vi "Image Measure_mag.vi"() -> ()   [LabVIEW 2016]
panel:
  in  "Magnification":dbl(ring) items=["0.78"=2.01724e-06, "1.0"=1.57574e-06, "1.25"=1.256e-06, "1.6"=9.82138e-07, "2.0"=7.83072e-07, "2.5"=6.26894e-07, "3.2"=4.92295e-07, "4.0"=3.93809e-07, "5.0"=3.15056e-07, "6.3"=2.59e-07, "8.0"=2.079e-07, "10.0"=1.646e-07, "12.5"=1.33e-07, "16.0"=1.02e-07]
  out "Line length":dbl format="%#_6pm"
  out "Line pixel length":dbl
  out "Line":T1 {"Start X" scale=0.0..1024.0; "End X" scale=0.0..1024.0}
  out "ROI":T2
  out "Tool":i32(ring) items=["None", "Selection Tool", "Point Tool", "Line Tool", "Rectangle Tool", "Oval Tool", "Polygon Tool", "ClosedFreehandTool", "Annulus Tool", "Rotated Rectangle Tool", "Zoom Tool", "Pan Tool", "Polyline Tool", "Freehand Tool"]
  out "Type":i32(ring) items=["No Event"=0, "Click Event"=1, "Draw Event"=2, "Size Event"=4, "Scroll Event"=5, "Double Click Event"=8]
  in  "Stop Button":bool
  in  "Image  path":path
  out "Image":T3(plugin-control)
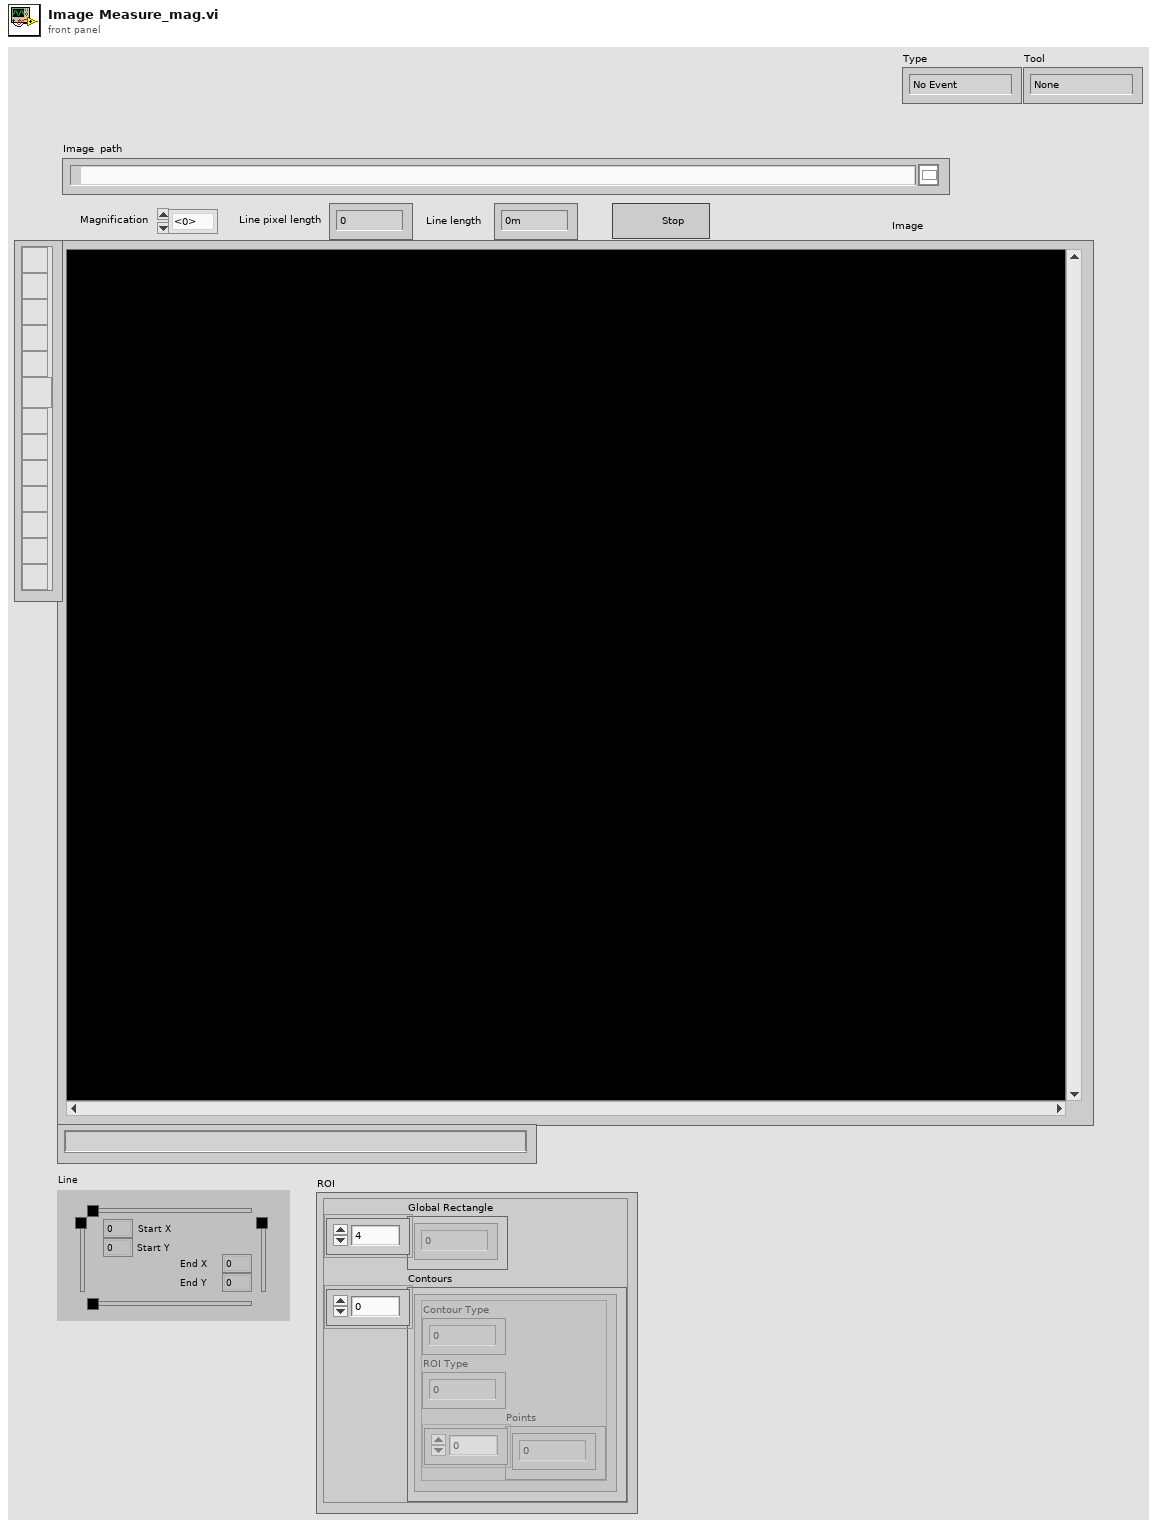
[diagram p1: front panel]
types:
  T1 = typedef "IMAQ Line" = cluster{"Start X":i32, "Start Y":i32, "End X":i32, "End Y":i32}
  T2 = cluster{"Global Rectangle":i32[], "Contours":cluster{"Contour Type":u32, "ROI Type":u32, "Points":i32[]}[]}
  T3 = typedef "IMAQ Image.ctl" = refnum<image>
  T4 = typedef "Image Type" = u32
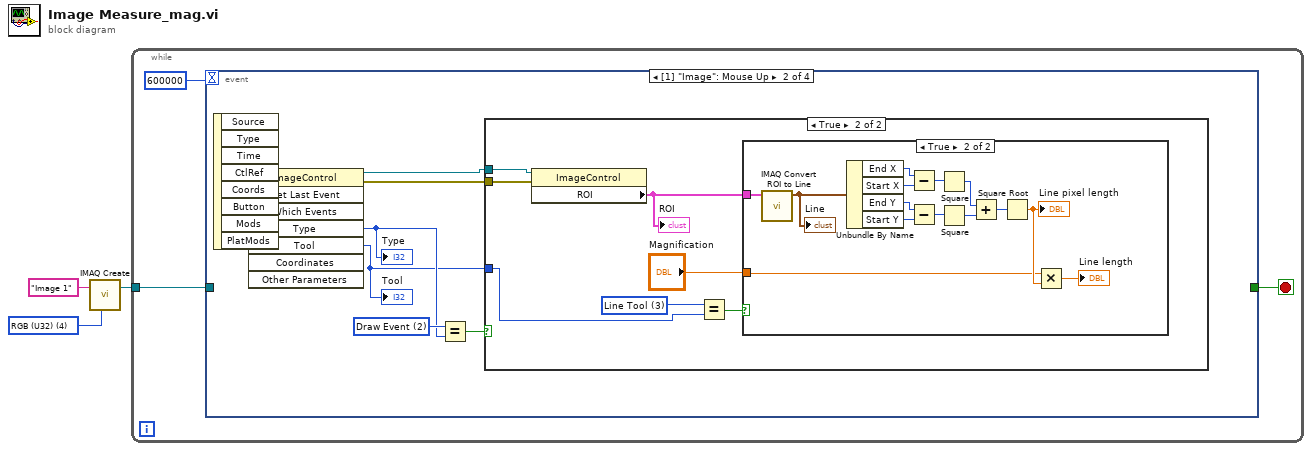
[diagram p0: block diagram]
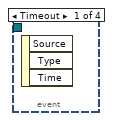
[diagram p2: hidden frame]
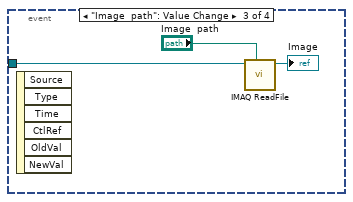
[diagram p5: hidden frame]
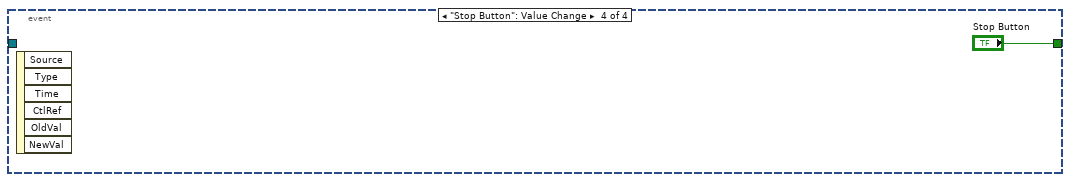
[diagram p6: hidden frame]
diagram:
  w2 = T4 4 items=["Grayscale (U8)", "Grayscale (I16)", "Grayscale (SGL)", "Complex (CSG)", "RGB (U32)", "HSL (U32)", "RGB (U64)", "Grayscale (U16)"] ("Image Type")
  n1 = call "IMAQ Create"("Image Name"="Image 1", "Image Type"=w2) -> ("New Image"=w1:T3)  [unwired: 3 in, 1 out]
  n2 = while {
    tunnel: w1 -> [w5]
    stop <- w6 stop-if-true
    n3 = event shown="[1] \"Image\": Mouse Up" {
      selector: _ -> [_ _ _ _]
      dyn-events: _ -> [_ _ _ _]
      timeout: 600000 -> [_ _ _ _]
      tunnel: [_ _ _ "Stop Button"] -> w6
      tunnel: w5 -> [_ _ w36 _]
      event Timeout {
        n4 = event-data() -> ()  [unwired: 1 in, 3 out]
      }
      event "Image": Mouse Up {
        w12 = 2 items=["No Event"=0, "Click Event"=1, "Draw Event"=2, "Size Event"=4, "Scroll Event"=5, "Double Click Event"=8] ("Type")
        n5 = event-data() -> ("CtlRef"=w13:refnum<vi>)  [unwired: 1 in, 7 out]
        n6 = invoke class="ImageControl" method="Get Last Event"(reference=w13) -> (reference out=w10:refnum<vi>, error out=w9:errorcluster, "Type"=w11:i32, "Tool"=w8:i32)  [unwired: 7 in, 4 out]
        "Type" <- w11
        "Tool" <- w8
        n7 = Equal?(x=w12, y=w11) -> (x = y?=w7:bool)
        n8 = case shown="True" w7 {
          tunnel: w10 -> [_ w20]
          tunnel: w9 -> [_ w19]
          tunnel: w8 -> [_ w14]
          frame False {
          }
          frame True {
            w15 = 3 items=["None", "Selection Tool", "Point Tool", "Line Tool", "Rectangle Tool", "Oval Tool", "Polygon Tool", "ClosedFreehandTool", "Annulus Tool", "Rotated Rectangle Tool", "Zoom Tool", "Pan Tool", "Polyline Tool", "Freehand Tool"] ("Tool")
            n9 = property class="ImageControl"(reference=w20, error in=w19) -> ("ROI"=w18:T2)  [unwired: 2 out]
            "ROI" <- w18
            n10 = Equal?(x=w15, y=w14) -> (x = y?=w16:bool)
            n11 = case shown="True" w16 {
              tunnel: w18 -> [_ w34]
              tunnel: "Magnification" -> [_ w21]
              frame False {
              }
              frame True {
                n12 = call "IMAQ Convert ROI to Line"("ROI Descriptor"=w34) -> ("Line"=w33:T1)  [unwired: 8 in, 1 out]
                "Line" <- w33
                n13 = Unbundle By Name(w33) -> ("End X"=w32:i32, "Start X"=w31:i32, "End Y"=w30:i32, "Start Y"=w29:i32)
                n14 = Subtract(x=w32, y=w31) -> (x-y=w28:i32)
                n15 = Subtract(x=w30, y=w29) -> (x-y=w27:i32)
                n16 = Square(x=w28) -> (x^2=w26:i32)
                n17 = Square(x=w27) -> (x^2=w25:i32)
                n18 = Add(x=w26, y=w25) -> (x+y=w24:i32)
                n19 = Square Root(x=w24) -> (sqrt(x)=w23:dbl)
                "Line pixel length" <- w23
                n20 = Multiply(x=w21, y=w23) -> (x*y=→"Line length":dbl)
              }
            }
          }
        }
      }
      event "Image  path": Value Change {
        n21 = event-data() -> ()  [unwired: 1 in, 6 out]
        n22 = call "IMAQ ReadFile"("File Path"="Image  path", "Image"=w36) -> ("Image Out"=→"Image":T3)  [unwired: 5 in, 4 out]
      }
      event "Stop Button": Value Change {
        n23 = event-data() -> ()  [unwired: 1 in, 6 out]
      }
    }
  }
